vi "Read Last Waveforms Means.vi"(8 "error in (no error)":errorcluster, 11 "Scope Base in":refnum<class "Scope Base.lvclass">) -> (0 "error out":errorcluster, 2 "Last Waveforms Means":map{u8, dbl}(c390), 3 "Scope Base out":refnum<class "Scope Base.lvclass">)   [LabVIEW 2023]
uses:
  Scope Base.lvclass
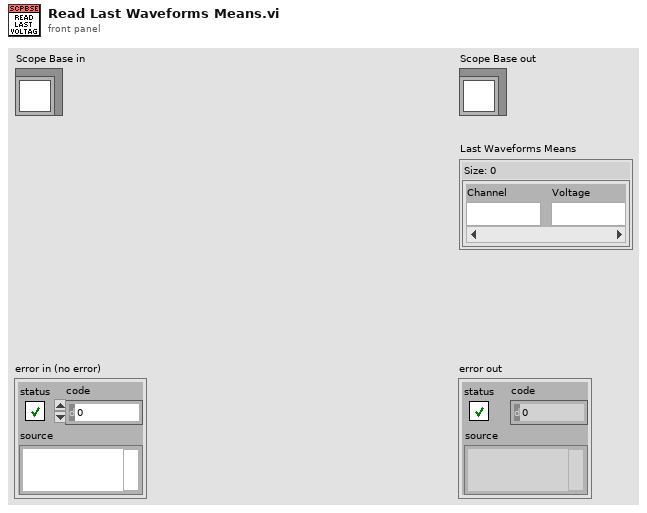
[diagram p1: front panel]
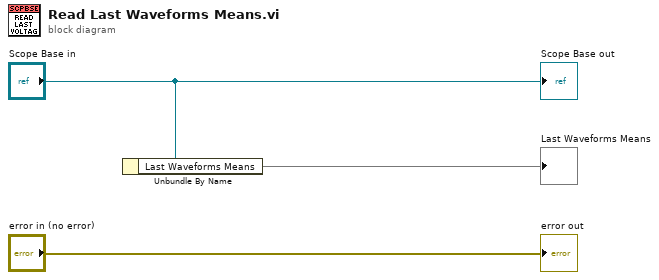
[diagram p0: block diagram]
diagram:
  n1 = Unbundle By Name("Scope Base in") -> ("Last Waveforms Means"=→"Last Waveforms Means")
  "error out" <- "error in (no error)"
  "Scope Base out" <- "Scope Base in"
